vi "Trigger.vi"(8 "error in (no error)":errorcluster, 11 "N5222A PNA in":refnum<class "N5222A PNA.lvclass">) -> (0 "error out":errorcluster, 3 "N5222A PNA out":refnum<class "N5222A PNA.lvclass">)   [LabVIEW 2018, in "N5222A PNA.lvclass"]
doc: "This VI checks the average count.\nThen it clears and restarts the average.\nThen it sends out as many single triggers as there are averages, so that it gets one full average and no more.\nThe manual recommends single trigger for sweep automation, so you are sure you have a whole sweep, or in this case sweeps."
uses:
  N5222A PNA.lvclass
panel:
  # "sens:swe:mode cont\n\nsens:swe:mode single"
  # "Need to do single and then wait for all averages to complete"
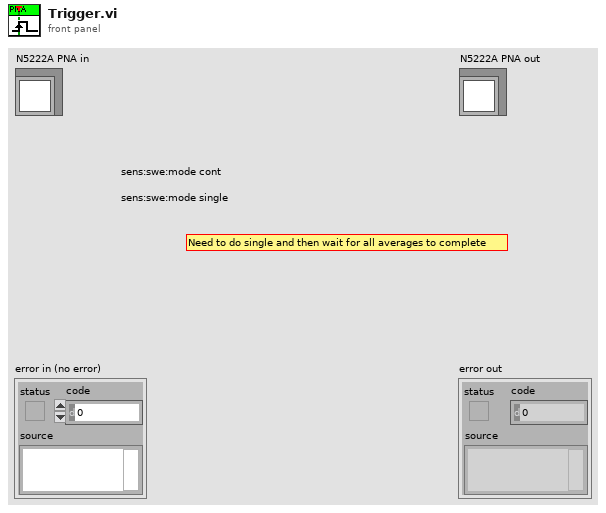
[diagram p1: front panel]
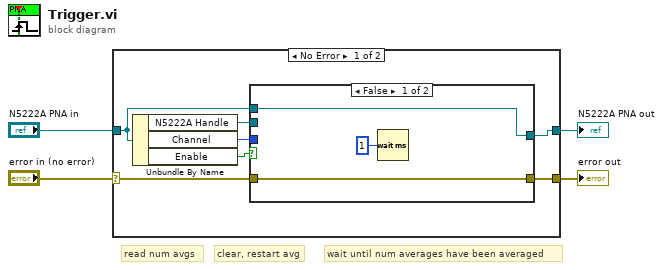
[diagram p0: block diagram]
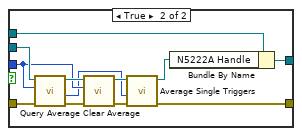
[diagram p2: hidden frame]
diagram:
  # "wait until num averages have been averaged"
  # "clear, restart avg"
  # "read num avgs"
  n1 = case shown="No Error" "error in (no error)" {
    selector: "error in (no error)" -> [w9 w28]
    tunnel: [w8 w28] -> w3
    tunnel: [w6 w27] -> w1
    tunnel: "N5222A PNA in" -> [w7 w27]
    frame No Error {
      n2 = Unbundle By Name(w7) -> ("N5222A Handle"=w11:refnum<visa-resource-name>, "Channel"=w10:i32, "Enable"=w5:bool)
      n3 = case shown="False" w5 {
        tunnel: w11 -> [_ w24]
        tunnel: w10 -> [_ w22]
        tunnel: w9 -> [w13 w20]
        tunnel: [w13 w18] -> w8
        tunnel: w7 -> [w14 w16]
        tunnel: [w14 w15] -> w6
        frame False {
          n4 = Wait (ms)(milliseconds to wait=u32 1) -> ()  [unwired: 1 out]
        }
        frame True {
          n5 = call "Query Average.vi"("Error In (no error)"=w20, "Channel (1)"=w22, "VISA Resource Name"=w24) -> ("Error Out"=w21:errorcluster, "Avg count"=w19:i32, "VISA Resource Name Out"=w23:refnum<visa-resource-name>)  [unwired: 6 in]
          n6 = call <instrlib>:"Clear Average.vi"("Error In (no error)"=w21, "Channel (1)"=w22, "VISA Resource Name"=w23) -> ("Error Out"=w26:errorcluster, "VISA Resource Name Out"=w25:refnum<visa-resource-name>)  [unwired: 7 in]
          n7 = call "Average Single Triggers.vi"("error in (no error)"=w26, "Average Count (1)"=w19, "VISA session"=w25) -> ("error out"=w18:errorcluster, "VISA session out"=w17:refnum<visa-resource-name>)  [unwired: 7 in]
          n8 = Bundle By Name(cluster=w16, "N5222A Handle"=w17) -> (w15:refnum<class "N5222A PNA.lvclass">)
        }
      }
    }
    frame Error {
    }
  }
  "error out" <- w3
  "N5222A PNA out" <- w1
